vi "Reset Timestamp.vi"(0 "fpga interface in":refnum<k20>, 11 "error in (no error)":errorcluster) -> (4 "fpga interface out":refnum<k20>, 15 "error out":errorcluster)   [LabVIEW 2023, in "GettingStarted_Acq_148X_Host.lvlib"]
uses:
  GettingStarted_Acq_148X_Host.lvlib
  Types/148x_Acq_FPGA_Reference.ctl
  <vilib>/Utility/error.llb/Error Cluster From Error Code.vi
  <vilib>/rvi/errors/niLvFpgaAdjustHostInterfaceError.vi
  <vilib>/rvi/interface/nirviReadWriteControl/nirviReadWriteControl.xnode
  NiFpgaLv.dll
  <vilib>/rvi/interface/Simulation/niFpgaSimulationCallBeginRW.vi
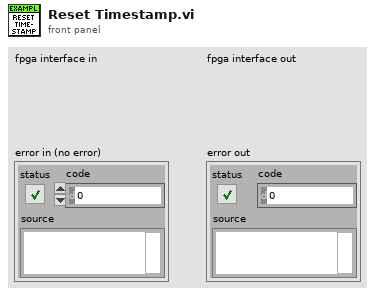
[diagram p1: front panel]
types:
  T1 = typedef "GettingStarted_Acq_148X_Host.lvlib/148x_Acq_FPGA_Reference.ctl" = refnum<k20>
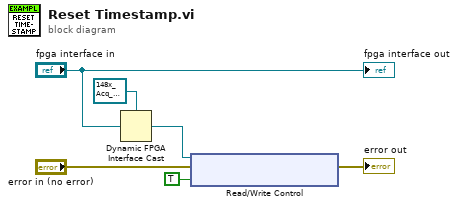
[diagram p0: block diagram]
diagram:
  n1 = Dynamic FPGA Interface Cast(Session In=T1 refnum ("FPGA VI Reference Out"), Type="fpga interface in") -> (Session Out=w4:T1)
  n2 = xnode "Read/Write Control"("FPGA VI Reference In"=w4, "error in"="error in (no error)", "reset timestamp (strobe)"=TRUE ("reset (strobe)")) -> ("error out"=→"error out":errorcluster)  [unwired: 1 out]
  "fpga interface out" <- "fpga interface in"
